vi "X轴回程连续扫描（1.0）.vi"(0 "VISA I":refnum<visa-resource-name>, 2 "X0":dbl, 3 "X":dbl, 4 "精度":dbl=0.001, 5 "细分设置":dbl=8.0, 6 "等待时间(ms)":u32=40, 7 "pulDDR2Length":u32, 8 "电机急停":bool, 9 "hDevice":i32, 11 "M-length":dbl, 13 "N-length":dbl) -> (14 "VISA O":refnum<visa-resource-name>, 15 "hDevice out":i32, 16 "X":dbl, 17 "强度图行":dbl[](array[numeric]), 18 "时域谱页":dbl[][](array[numeric]), 19 "幅频谱页":dbl[][](array[numeric]))   [LabVIEW 2016]
panel:
  out "大小":i32[](array[numeric])
  out "幅频谱":dbl[](graph)
  out "时域谱":dbl[](graph)
  # "X："
  # "时域谱"
  # "频域谱"
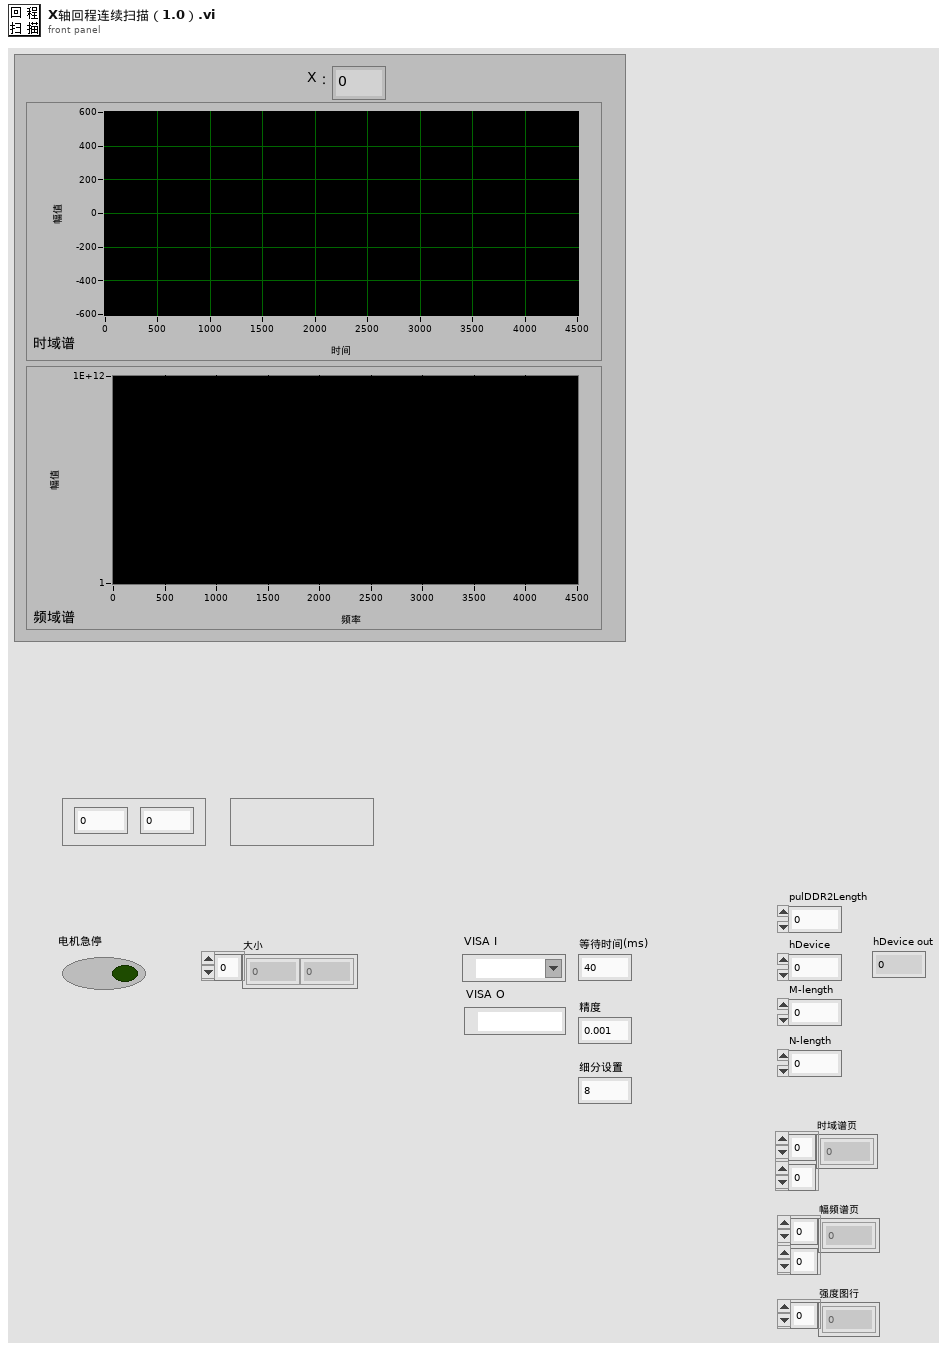
[diagram p1: front panel]
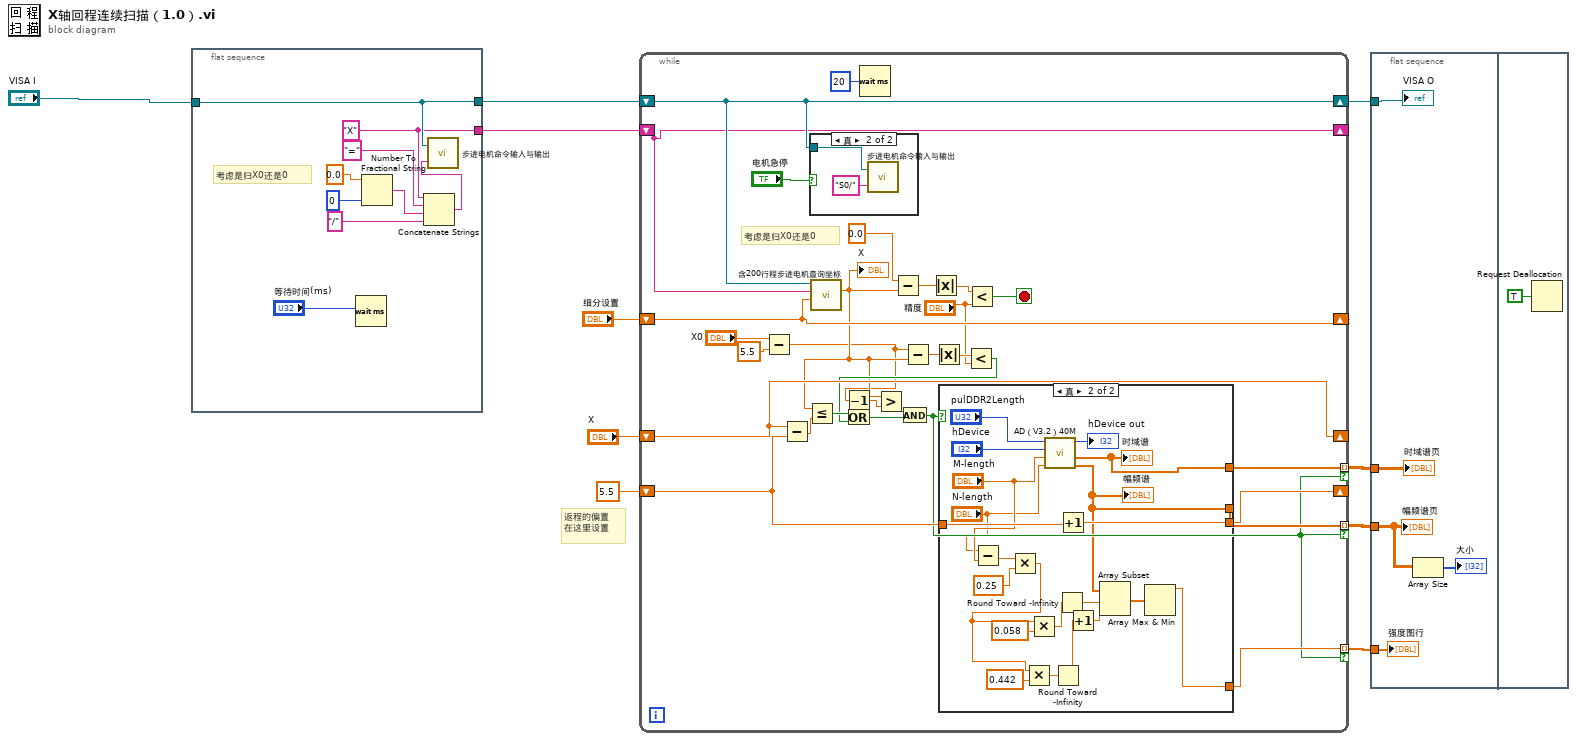
[diagram p0: block diagram]
diagram:
  # "返程的偏置\n在这里设置"
  n1 = flat-sequence {
    tunnel: "VISA I" -> [w14]
    tunnel: [w14] -> w9
    tunnel: [w13] -> w8
    frame #0 {
      w13 = "X"
      # "考虑是归X0还是0"
      n2 = Wait (ms)(milliseconds to wait="等待时间(ms)") -> ()  [unwired: 1 out]
      n3 = Number To Fractional String(number=0.0 ("x"), precision (6)=i16 0 ("精度(6)")) -> (F-format string=w18:string)  [unwired: 2 out]
      n4 = Concatenate Strings(w13, "=" ("字符串"), w18, "/" ("字符串")) -> (w15:string)
      n5 = call "步进电机命令输入与输出.vi"("输入字符串"=w15, "串口通信端口"=w14) -> ()  [unwired: 1 out]
    }
  }
  n6 = while {
    shift-right: [w46] -> w3
    shift-left: w9 -> [w46]
    shift-right: [w34] -> _
    shift-left: "X" -> [w34]
    shift-right: [w42] -> _
    shift-left: "细分设置" -> [w42]
    shift-right: [w36] -> _
    shift-left: w8 -> [w36]
    tunnel: [w41] -> w4 mode=indexing if=w27
    shift-right: [w35] -> _
    shift-left: 5.5 -> [w40]
    tunnel: [w39] -> w6 mode=indexing if=w27
    tunnel: [w38] -> w5 mode=indexing if=w27
    stop <- w37 stop-if-true
    # "考虑是归X0还是0"
    n7 = Subtract(x="X0", y=5.5) -> (x-y=w21:dbl)
    n8 = Subtract(x=w34, y=w40) -> (x-y=w43:dbl)
    n9 = case shown="真" "电机急停" {
      tunnel: w46 -> [_ w71]
      frame False {
      }
      frame True {
        n10 = call "步进电机命令输入与输出.vi"("输入字符串"="S0/", "串口通信端口"=w71) -> ()  [unwired: 1 out]
      }
    }
    n11 = call "含200行程步进电机查询坐标.vi"("细分设置"=w42, "查询坐标轴"=w36, "串口通信端口"=w46) -> ("坐标(mm)"=w23:dbl)  [unwired: 8 in]
    "X" <- w23
    n12 = Less Or Equal?(x=w23, y=w43) -> (x <= y?=w32:bool)
    n13 = Decrement(x=w21) -> (x-1=w24:dbl)
    n14 = Wait (ms)(milliseconds to wait=u32 20 ("等待时间（毫秒）")) -> ()  [unwired: 1 out]
    n15 = Greater?(x=w23, y=w24) -> (0:w26:bool)
    n16 = Subtract(x=0.0, y=w23) -> (x-y=w48:dbl)
    n17 = Subtract(x=w21, y=w23) -> (x-y=w30:dbl)
    n18 = Absolute Value(x=w48) -> (abs(x)=w47:dbl)
    n19 = Absolute Value(x=w30) -> (abs(x)=w31:dbl)
    n20 = Less?(x=w31, y="精度") -> (x < y?=w28:bool)
    n21 = Or(x=w32, y=w28) -> (x .or. y?=w25:bool)
    n22 = And(x=w26, y=w25) -> (x .and. y?=w27:bool)
    n23 = case shown="真" w27 {
      tunnel: [_ w51] -> w41
      tunnel: w40 -> [w49 w67]
      tunnel: [w49 w66] -> w35
      tunnel: [_ w65] -> w39
      tunnel: [_ w50] -> w38
      frame False {
      }
      frame True {
        n24 = Subtract(x="N-length", y="M-length") -> (x-y=w63:dbl)
        n25 = Multiply(x=w63, y=0.25) -> (x*y=w53:dbl)
        n26 = Multiply(x=w53, y=0.442) -> (x*y=w56:dbl)
        n27 = Multiply(x=w53, y=0.058) -> (x*y=w58:dbl)
        n28 = call "AD（V3.2）40M.vi"("N-length"="N-length", "M-length"="M-length", "hDevice"="hDevice", "pulDDR2Length"="pulDDR2Length") -> ("幅频谱"=w51:dbl[], "时域谱"=w65:dbl[], "hDevice out"=→"hDevice out":i32)  [unwired: 5 in]
        "时域谱" <- w65
        "幅频谱" <- w51
        n29 = Round Toward -Infinity(1:w56) -> (0:w54:dbl)
        n30 = Round Toward -Infinity(1:w58) -> (0:w57:dbl)
        n31 = Increment(x=w67) -> (x+1=w66:dbl)
        n32 = Increment(x=w54) -> (x+1=w60:dbl)
        n33 = Array Subset(array=w51, index=w57, length=w60) -> (w52:dbl[])
        n34 = Array Max & Min(array=w52) -> (max value=w50:dbl)  [unwired: 3 out]
      }
    }
    n35 = Less?(x=w47, y="精度") -> (x < y?=w37:bool)
  }
  n36 = flat-sequence {
    tunnel: w6 -> [w77]
    tunnel: w5 -> [w76]
    tunnel: w4 -> [w75]
    tunnel: w3 -> [w73]
    frame #0 {
      n37 = Array Size(array=w75) -> (size(s)=→"大小":i32[])
      "VISA O" <- w73
      "幅频谱页" <- w75
      "时域谱页" <- w77
      "强度图行" <- w76
    }
    frame #1 {
      n38 = Request Deallocation(TRUE ("标志")) -> ()
    }
  }
